vi "Lookup Double Channel.vi"(8 "error in (no error)":errorcluster, 10 "Channel Name":string, 11 "ChannelService in":refnum<class "ChannelService.lvclass">) -> (0 "error out":errorcluster, 2 "Channel":refnum<class "Channel DBL.lvclass">, 3 "ChannelService out":refnum<class "ChannelService.lvclass">)   [LabVIEW 2020, in "Vecto.lvlib" / "ChannelService.lvclass"]
uses:
  ChannelService.lvclass
  Channel DBL/Channel DBL.lvclass
  ChannelValue/DoubleChannelValue.lvclass
  Lookup Channel Data.ctl
  lv-promises/Promises/Promise/Promise.lvclass
  Group Data Type.ctl
  ChannelService.lvclass/ChannelService.ctl
  lv-promises/Promises/Promise/Promise.lvclass/Promise.ctl
  lv-promises/Promises/Future/Future.lvclass/Future.ctl
  ChannelValue/DoubleChannelValue.lvclass/DoubleChannelValue.ctl
  lv-promises/Promises/Future/Future.lvclass
  VectoConfig/VectoConfig.lvlib
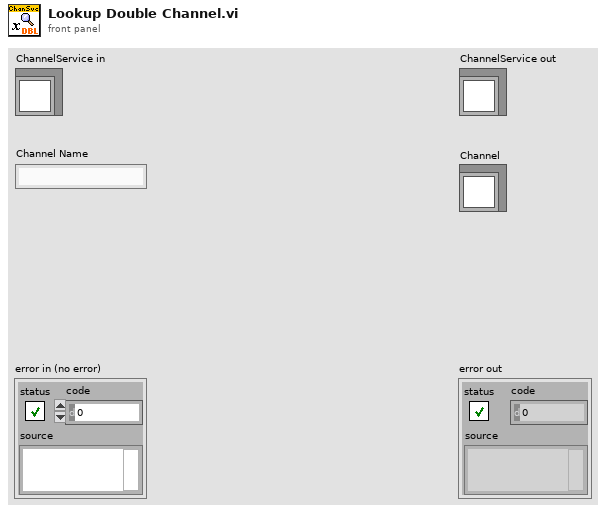
[diagram p1: front panel]
types:
  T1 = typedef "VectoConfig.lvlib/Group Data Type.ctl" = enum16{"Double", "String", "Bool"}
  T2 = typedef "Vecto.lvlib/ChannelService.lvclass/Lookup Channel Data.ctl" = cluster{"Channel Name":string, "Promise":refnum<class "Promise.lvclass">, "Data Type":T1}
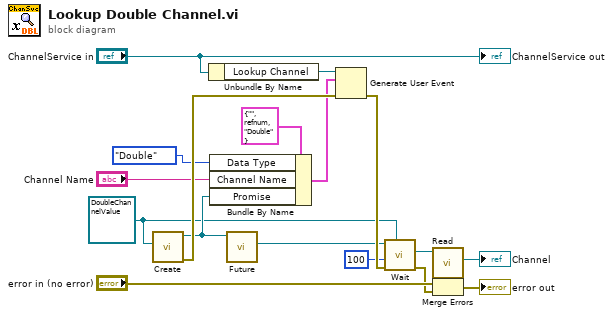
[diagram p0: block diagram]
diagram:
  w5 = refnum<class "DoubleChannelValue.lvclass"> refnum ("Vecto.lvlib:ChannelValue.lvclass")
  n1 = call "Create.vi"("Result Type (None)"=w5) -> ("error out"=w16:errorcluster, "Promise"=w13:refnum<class "Promise.lvclass">)  [unwired: 9 in]
  n2 = Unbundle By Name("ChannelService in") -> ("Lookup Channel"=w10:refnum<user-event>)
  n3 = Bundle By Name(cluster=T2 {"Channel Name"="", "Promise"=refnum, "Data Type"=enum."Double"} ("Lookup Channel Data"), "Data Type"=Group_Data_Type."Double", "Channel Name"="Channel Name", "Promise"=w13) -> (w9:T2)
  n4 = call "Future.vi"("Promise in"=w13) -> ("Future"=w8:refnum<class "Future.lvclass">)  [unwired: 9 in, 1 out]
  n5 = Generate User Event(user event=w10, event data cluster=w9, error in=w16) -> (error out=w17:errorcluster)  [unwired: 1 in, 1 out]
  n6 = call "Wait.vi"("Result Type (None)"=w5, "error in (no error)"=w17, "Timeout mS (-1)"=100, "Future in"=w8) -> ("error out"=w2:errorcluster, "Result"=w6:refnum<class "DoubleChannelValue.lvclass">)  [unwired: 6 in]
  n7 = call "Read.vi"("ChannelValue in"=w6) -> ("Channel"=→"Channel":refnum<class "Channel DBL.lvclass">)  [unwired: 10 in]
  n8 = Merge Errors("error in (no error)", w2) -> (→"error out":errorcluster)
  "ChannelService out" <- "ChannelService in"
